vi "CPP-FIDpulseResponse.vi"() -> (5 "Plug in titles":string[](array[string]), 7 "Plug in values":string[](array[string]))   [LabVIEW 2021]
uses:
  Globals/Meas_global.vi
  <vilib>/measure/NI_MAPro.lvlib
  <vilib>/measure/mascope.llb/Transition Measurements N chan.vi
  <vilib>/measure/mascope.llb/Pulse Measurements N chan.vi
  <vilib>/Waveform/WDTOps.llb/WDT Get Waveform Subset DBL.vi
  <vilib>/measure/mascope.llb/Amplitude and Levels N chan.vi
  <vilib>/Analysis/NI_AALBase.lvlib
  <vilib>/Analysis/baseanly.llb/Mean (DBL).vi
panel:
  out "Cropped Means":dbl[](array[numeric])
  out "Cropped Sum all graph":waveform(dbl)[](graph)
  out "Duration of pulses":dbl
  out "Cropped Sum(all)":dbl[](array[numeric]) format="%#.0f"
  out "Starts":dbl[](array[numeric])
  out "sum(all)":dbl[](array[numeric])
  out "names":string[](array[string])
  out "NupEdges":i16[](array[numeric])
  out "sum(90-90)":dbl[](array[numeric])
  out "sum(10-10)":dbl[](array[numeric])
  out "(90-90) Graph":waveform(dbl)[](graph)
  out "(10-10) Graph":waveform(dbl)[](graph)
  out "t(90-90)":dbl[](array[numeric]) format="%.1f"
  out "t(10-10)":dbl[](array[numeric]) format="%.1f"
  out "complete":dbl[](array[numeric])
  out "t(10)":dbl[](array[numeric]) format="%.2f"
  out "slope (ppm/s)":dbl[](array[numeric]) format="%_3f"
  out "t(90)":dbl[](array[numeric]) format="%.2f"
  out "period (s)":dbl[](array[numeric]) format="%.1f"
  out "pulse duration (s)":dbl[](array[numeric]) format="%.1f"
  out "amplitude (ppm)":dbl[](array[numeric]) format="%.3f"
  in  "Enum":enum16{"Eng Units", "Voltages"}(ring)
  out "XY Graph":cluster{"Time (s)":dbl[], "Voltage":dbl[]}[](graph)
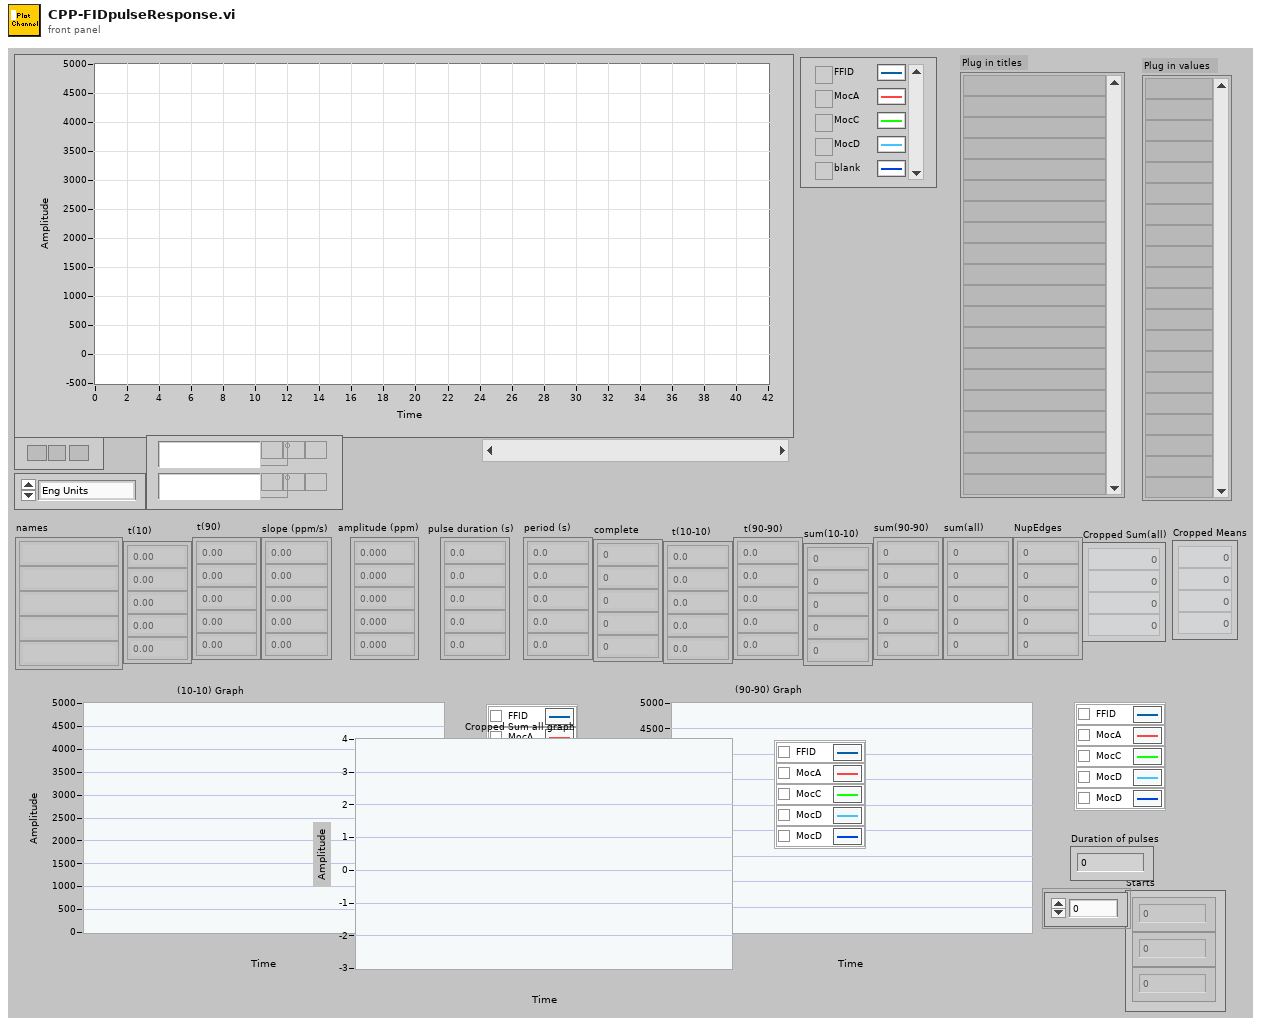
[diagram p1: front panel]
types:
  T1 = cluster{"method":enum32{"histogram", "peak", "auto select"}, "histogram size":i32, "histogram method":enum16{"mode"}, "reserved":dbl}
  T2 = cluster{"high ref level":dbl, "mid ref level":dbl, "low ref level":dbl, "ref units":u16}
  T3 = typedef "Analysis_info_cluster.ctl" = cluster{"Colour":u32, "Inst type":T4, "Inst name":string, "Symbol":string, "Code name":string, "Extra Info":string, "Inst Array":T5, "Extra Titles":string[], "Extra Values":string[], "U":dbl, "u^2":dbl, "u^3":dbl, "u^4":dbl, "Skew_u":dbl, "Kurt_u":dbl, "Sd Error in Mean":dbl, "% u'/U":dbl, "X":dbl, "Y":dbl, "Z":dbl, "Timescale integral Estimate":dbl, "Sd Error in Variance":dbl, "Calib File":path, "Calib Constants":dbl[], "Output Position":bool, "Stats":enum16{"None", "Basic", "Full"}, "Av Sampling Rate":dbl, "Av No of Samples":dbl, "Total Meas Time (s)":dbl, "ADAM Ch Name":string, "Max value":dbl, "Min value":dbl, "Req Sample Rate Hz":dbl, "Sync Delay Time (s)":dbl, "Ch No":i16, "Device":string, "Use Latest Calib":bool, "Port":string, "Metadata Ch Names":string[], "Metadata Ch Values":string[], "Label":string}
  T4 = typedef "Inst_type.ctl" = enum16{"Raw voltage", "Raw with zero offsetting", "Propeller anemometer", "Pressure Transducer", "Pitot-static tube", "Hot wire", "Cross wire 1", "Cross wire 2", "Generic Linear", "Generic Polynomial", "Generic BackPoly", "Fast FID", "Thermocouple", "Cold wire", "Pulsed Wire", "LDA Vel", "LDA Tran time", "LDA Arr time", "Microphone"}
  T5 = typedef "Instrument_Array.ctl" = enum16{"PWA", "LDA", "Analogue"}
  T6 = typedef "Time_Trace_Cluster.ctl" = cluster{"Weighting":dbl[], "Voltage":dbl[], "Eng Values":dbl[]}
  T7 = cluster{"start time":dbl, "end time":dbl, "ref levels":cluster{"high ref level":dbl, "mid ref level":dbl, "low ref level":dbl, "ref units":u16}}[]
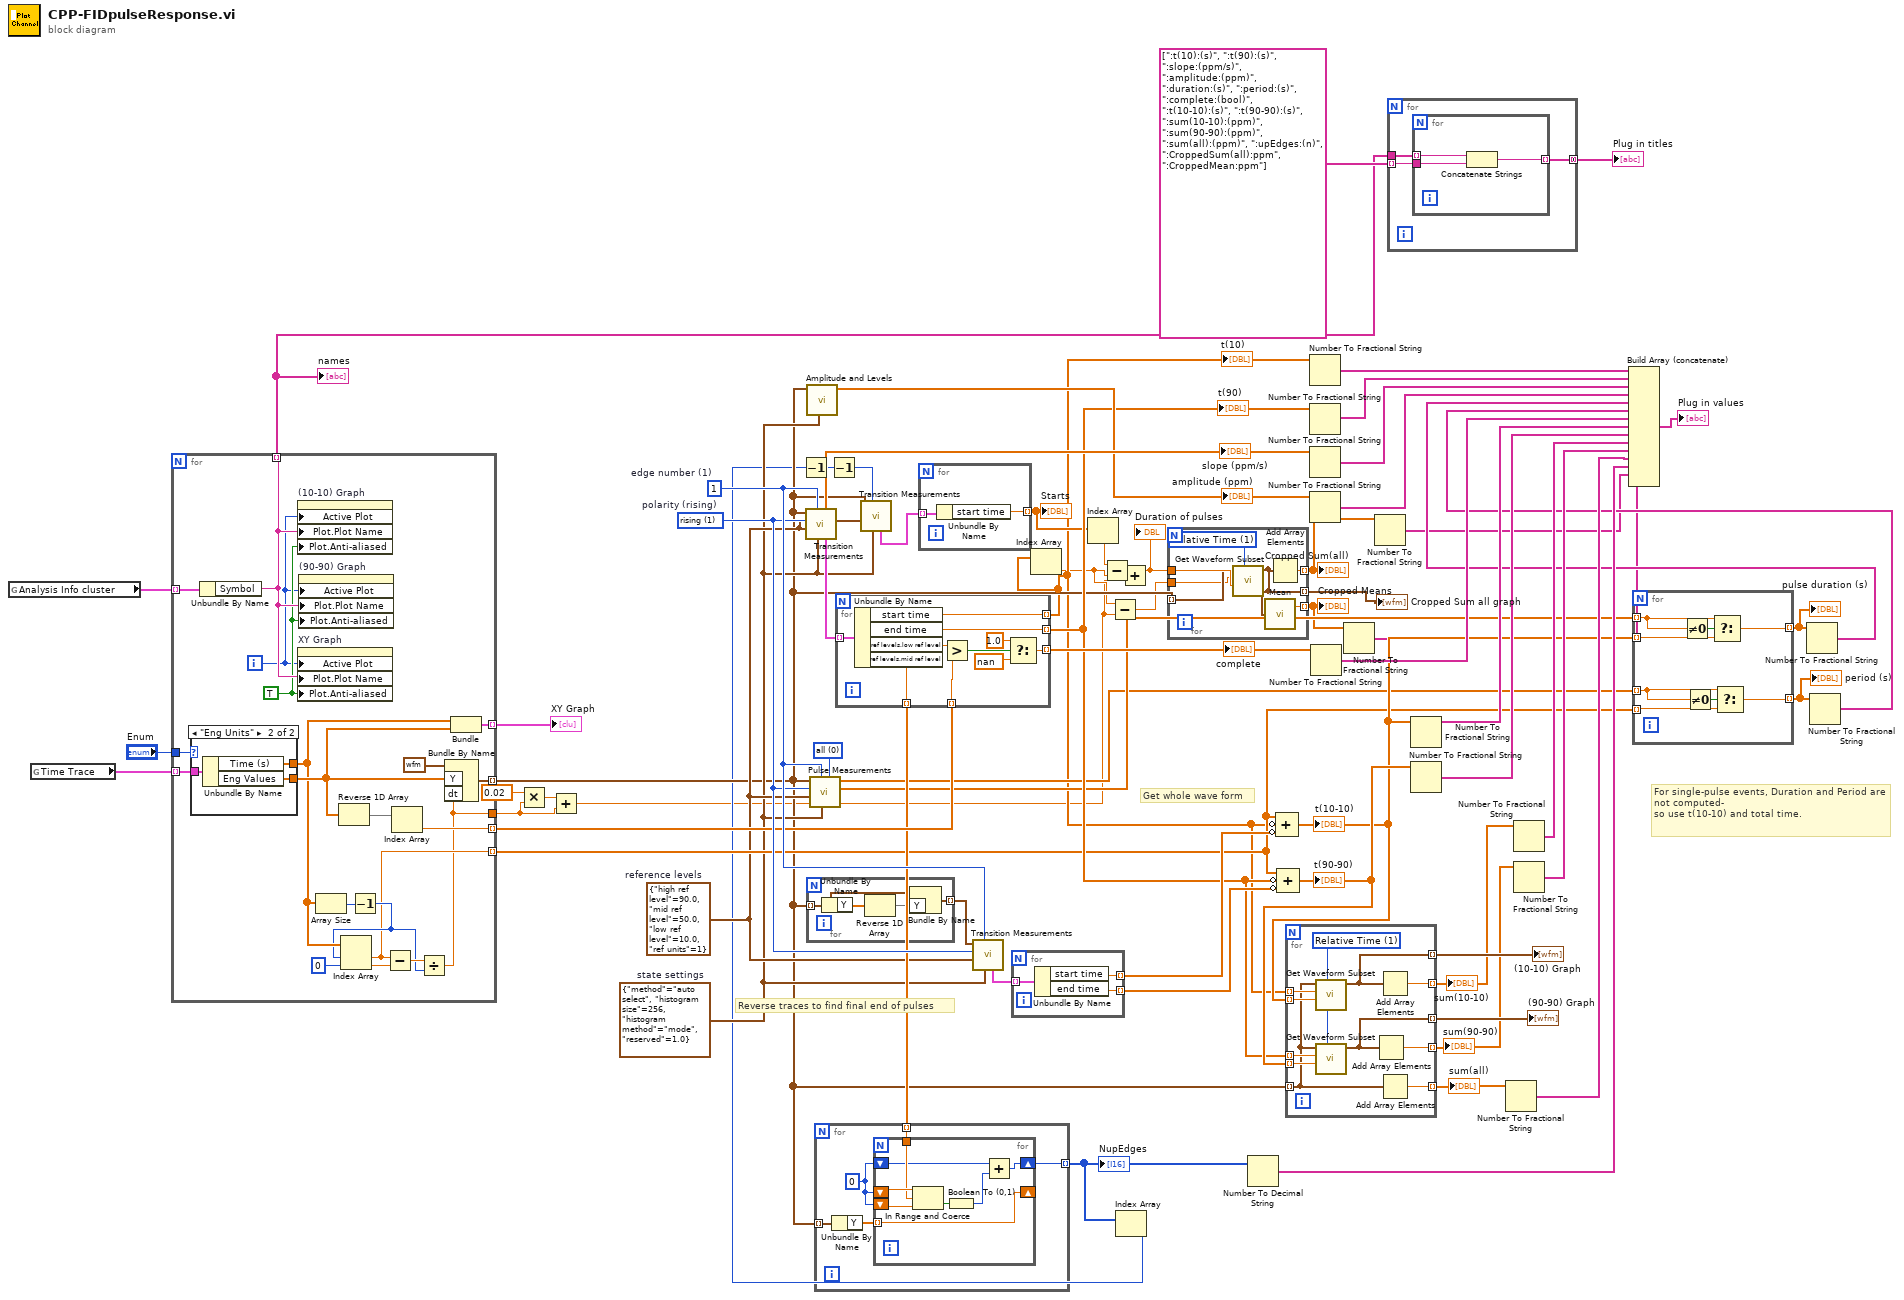
[diagram p0: block diagram]
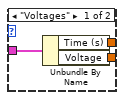
[diagram p2: hidden frame]
diagram:
  w54 = 1  # edge number (1)
  w53 = u16 1 items=["falling", "rising"]  # polarity (rising)
  w23 = T1 {"method"=enum."auto select", "histogram size"=256, "histogram method"=enum."mode", "reserved"=1.0}  # state settings
  w24 = T2 {"high ref level"=90.0, "mid ref level"=50.0, "low ref level"=10.0, "ref units"=1}  # reference levels
  w67 = u16 0 items=["all", "no period and duty cycle"] ("export mode")
  # "Get whole wave form"
  # "For single-pulse events, Duration and Period are not computed-\nso use t(10-10) and total time."
  # "Reverse traces to find final end of pulses"
  n1 = global read "Meas_global.vi" "Analysis Info cluster"() -> (w70:T3[])
  n2 = global read "Meas_global.vi" "Time Trace"() -> (w71:T6[])
  n3 = for {
    tunnel: w71 -> [w91] mode=indexing
    tunnel: [w90] -> w68 mode=indexing
    tunnel: w70 -> [w89] mode=indexing
    tunnel: "Enum" -> [w88]
    tunnel: [w87] -> w20 mode=indexing
    tunnel: [w76] -> w36 mode=indexing
    tunnel: [w84] -> w49 mode=indexing
    tunnel: [w77] -> w29 mode=indexing
    tunnel: [w72] -> w4
    i -> [w74]
    w75 = TRUE ("Plot.Anti-aliased")
    n4 = case shown="\"Eng Units\"" w88 {
      tunnel: [w94 w97] -> w85
      tunnel: [w93 w96] -> w82
      tunnel: w91 -> [w92 w95]
      frame "Voltages" {
        n5 = Unbundle By Name(w92) -> ("Time (s)"=w93:dbl[], "Voltage"=w94:dbl[])
      }
      frame "Eng Units" {
        n6 = Unbundle By Name(w95) -> ("Time (s)"=w96:dbl[], "Eng Values"=w97:dbl[])
      }
    }
    n7 = Unbundle By Name(w89) -> ("Symbol"=w76:string)
    n8 = property on="(10-10) Graph" class="WFGraph (strict)"("Active Plot"=w74, "Plot.Plot Name"=w76, "Plot.Anti-aliased"=w75) -> ()  [unwired: 2 in, 2 out]
    n9 = property on="XY Graph" class="XYGraph (strict)"("Active Plot"=w74, "Plot.Plot Name"=w76, "Plot.Anti-aliased"=w75) -> ()  [unwired: 2 in, 2 out]
    n10 = property on="(90-90) Graph" class="WFGraph (strict)"("Active Plot"=w74, "Plot.Plot Name"=w76, "Plot.Anti-aliased"=w75) -> ()  [unwired: 2 in, 2 out]
    n11 = Array Size(array=w82) -> (size(s)=w81:i32)
    n12 = Reverse 1D Array(array=w85) -> (reversed array=w86:dbl[])
    n13 = Decrement(x=w81) -> (x-1=w78:i32)
    n14 = Index Array(array=w82, index #1=w78, index #2=0 ("index")) -> (element #1=w77:dbl, element #2=w80:dbl)
    n15 = Subtract(x=w77, y=w80) -> (x-y=w83:dbl)
    n16 = Index Array(array=w86) -> (element=w84:dbl)  [unwired: 1 in]
    n17 = Divide(x=w83, y=w78) -> (x/y=w72:dbl)
    n18 = Bundle By Name(cluster=waveform(dbl) {"t0"=timestamp(0 s since 1904-01-01), "dt"=1.0, "Y"=[]} ("waveform"), "Y"=w85, "dt"=w72) -> (w87:waveform(dbl))
    n19 = Bundle("Time (s)"=w82, "Eng Values"=w85) -> (w90:cluster{"Time (s)":dbl[], "Eng Values":dbl[]})  [unwired: 1 in]
  }
  "XY Graph" <- w68
  "names" <- w36
  n20 = Multiply(x=0.02, y=w4) -> (x*y=w2:dbl)
  n21 = Add(x=w2, y=w4) -> (x+y=w1:dbl)
  n22 = call-poly <vilib>:"Transition Measurements.vi"("percent level settings"=w23, "edge number (1)"=w54, "reference levels"=w24, "polarity (rising)"=w53, "signal(s) in"=w20) -> ("measurement info"=w66:T7, "slope"=w61:dbl[])  [unwired: 1 in, 4 out]
  "slope (ppm/s)" <- w61
  n23 = call-poly <vilib>:"Amplitude and Levels.vi"("state settings"=w23, "signal(s) in"=w20) -> ("amplitude"=w58:dbl[])  [unwired: 6 in, 3 out]
  "amplitude (ppm)" <- w58
  n24 = for {
    tunnel: w20 -> [w98] mode=indexing
    tunnel: [w100] -> w52 mode=indexing
    n25 = Unbundle By Name(w98) -> ("Y"=w101:dbl[])
    n26 = Reverse 1D Array(array=w101) -> (reversed array=w99:dbl[])
    n27 = Bundle By Name(cluster=w98, "Y"=w99) -> (w100:waveform(dbl))
  }
  n28 = call-poly <vilib>:"Pulse Measurements.vi"("export mode"=w67, "percent level settings"=w23, "pulse number (1)"=w54, "reference levels"=w24, "polarity (high)"=w53, "signal(s) in"=w20) -> ("pulse duration"=w32:dbl[], "period"=w27:dbl[])  [unwired: 1 in, 3 out]
  n29 = for {
    tunnel: w66 -> [w111] mode=indexing
    tunnel: w49 -> [w106] mode=indexing
    tunnel: [w108] -> w56 mode=indexing
    tunnel: [w104] -> w40 mode=indexing
    tunnel: [w103] -> w17 mode=indexing
    tunnel: [w102] -> w37 mode=indexing
    n30 = Unbundle By Name(w111) -> ("start time"=w103:dbl, "end time"=w104:dbl, "ref levels.low ref level"=w110:dbl, "ref levels.mid ref level"=w102:dbl)
    n31 = Greater?(x=w110, y=w106) -> (0:w109:bool)
    n32 = Select(t=1.0, s=w109, f=nan) -> (s? t:f=w108:dbl)
  }
  "t(90)" <- w40
  "t(10)" <- w17
  "complete" <- w56
  n33 = for {
    tunnel: w20 -> [w113] mode=indexing
    tunnel: w37 -> [w116] mode=indexing
    tunnel: [w115] -> w16 mode=indexing
    w114 = i16 0
    n34 = Unbundle By Name(w113) -> ("Y"=w112:dbl[])
    n35 = for {
      shift-right: [w117] -> _
      shift-left: w114 -> [w124]
      shift-left: w114 -> [w123]
      tunnel: w116 -> [w122]
      shift-right: [w120] -> w115
      shift-left: w114 -> [w118]
      tunnel: w112 -> [w117] mode=indexing
      n36 = In Range and Coerce(upper limit=w124, x=w122, lower limit=w123) -> (In Range?=w121:bool)  [unwired: 1 out]
      n37 = Boolean To (0,1)(Boolean=w121) -> (0, 1=w119:i16)
      n38 = Add(x=w118, y=w119) -> (x+y=w120:i16)
    }
  }
  "NupEdges" <- w16
  n39 = call-poly <vilib>:"Transition Measurements.vi"("percent level settings"=w23, "edge number (1)"=w54, "reference levels"=w24, "polarity (rising)"=w53, "signal(s) in"=w52) -> ("measurement info"=w51:T7)  [unwired: 1 in, 5 out]
  n40 = for {
    tunnel: w51 -> [w127] mode=indexing
    tunnel: [w126] -> w50 mode=indexing
    tunnel: [w125] -> w48 mode=indexing
    n41 = Unbundle By Name(w127) -> ("start time"=w125:dbl, "end time"=w126:dbl)
  }
  n42 = Index Array(array=w17) -> (element=w13:dbl)  [unwired: 1 in]
  n43 = Subtract(x=w13, y=w1) -> (x-y=w12:dbl)
  n44 = Index Array(array=w16) -> (element=w15:i16)  [unwired: 1 in]
  n45 = Decrement(x=w15) -> (x-1=w8:i16)
  n46 = Decrement(x=w8) -> (x-1=w9:i16)
  n47 = call-poly <vilib>:"Transition Measurements.vi"("percent level settings"=w23, "edge number (1)"=w9, "reference levels"=w24, "signal(s) in"=w20) -> ("measurement info"=w22:T7)  [unwired: 2 in, 5 out]
  n48 = for {
    tunnel: w22 -> [w129] mode=indexing
    tunnel: [w128] -> w19 mode=indexing
    n49 = Unbundle By Name(w129) -> ("start time"=w128:dbl)
  }
  "Starts" <- w19
  n50 = Index Array(array=w19) -> (element=w18:dbl)  [unwired: 1 in]
  n51 = Subtract(x=w18, y=w13) -> (x-y=w21:dbl)
  n52 = Add(x=w21, y=w1) -> (x+y=w7:dbl)
  "Duration of pulses" <- w7
  n53 = for {
    tunnel: w7 -> [w136]
    tunnel: w20 -> [w135] mode=indexing
    tunnel: [w134] -> w11 mode=indexing
    tunnel: w12 -> [w133]
    tunnel: [w131] -> w14 mode=indexing
    tunnel: [w130] -> w6 mode=indexing
    w132 = u16 1 items=["Samples", "Relative Time"] ("start/duration format")
    n54 = call-poly <vilib>:"Get Waveform Subset.vi"("start/duration format"=w132, "duration"=w136, "start samples/time"=w133, "waveform in"=w135) -> ("waveform out"=w131:waveform(dbl))  [unwired: 2 in, 3 out]
    n55 = call-poly <vilib>:"Mean.vi"("X"=w131) -> ("mean"=w130:dbl)  [unwired: 1 out]
    n56 = Add Array Elements(numeric array=w131) -> (sum=w134:dbl)
  }
  "Cropped Sum(all)" <- w11
  "Cropped Sum all graph" <- w14
  "Cropped Means" <- w6
  n57 = Number To Decimal String(number=w16) -> (decimal integer string=w35:string[])  [unwired: 1 in]
  n58 = Compound Arithmetic op=ADD(w29, invert w17, invert w48) -> (w31:dbl[])
  "t(10-10)" <- w31
  n59 = Compound Arithmetic op=ADD(w29, invert w40, invert w50) -> (w47:dbl[])
  "t(90-90)" <- w47
  n60 = for {
    tunnel: w17 -> [w147] mode=indexing
    tunnel: w20 -> [w138] mode=indexing
    tunnel: w40 -> [w146] mode=indexing
    tunnel: w47 -> [w145] mode=indexing
    tunnel: w31 -> [w144] mode=indexing
    tunnel: [w142] -> w42 mode=indexing
    tunnel: [w140] -> w41 mode=indexing
    tunnel: [w141] -> w39 mode=indexing
    tunnel: [w139] -> w38 mode=indexing
    tunnel: [w137] -> w34 mode=indexing
    w143 = u16 1 items=["Samples", "Relative Time"] ("start/duration format")
    n61 = call-poly <vilib>:"Get Waveform Subset.vi"("start/duration format"=w143, "duration"=w144, "start samples/time"=w147, "waveform in"=w138) -> ("waveform out"=w142:waveform(dbl))  [unwired: 2 in, 3 out]
    n62 = call-poly <vilib>:"Get Waveform Subset.vi"("start/duration format"=w143, "duration"=w145, "start samples/time"=w146, "waveform in"=w138) -> ("waveform out"=w140:waveform(dbl))  [unwired: 2 in, 3 out]
    n63 = Add Array Elements(numeric array=w140) -> (sum=w139:dbl)
    n64 = Add Array Elements(numeric array=w142) -> (sum=w141:dbl)
    n65 = Add Array Elements(numeric array=w138) -> (sum=w137:dbl)
  }
  "(10-10) Graph" <- w42
  "(90-90) Graph" <- w41
  "sum(10-10)" <- w39
  "sum(90-90)" <- w38
  "sum(all)" <- w34
  n66 = Number To Fractional String(number=w17) -> (F-format string=w63:string[])  [unwired: 3 in]
  n67 = Number To Fractional String(number=w40) -> (F-format string=w60:string[])  [unwired: 3 in]
  n68 = Number To Fractional String(number=w61) -> (F-format string=w59:string[])  [unwired: 3 in]
  n69 = Number To Fractional String(number=w58) -> (F-format string=w57:string[])  [unwired: 3 in]
  n70 = Number To Fractional String(number=w56) -> (F-format string=w55:string[])  [unwired: 3 in]
  n71 = Number To Fractional String(number=w6) -> (F-format string=w5:string[])  [unwired: 3 in]
  n72 = Number To Fractional String(number=w11) -> (F-format string=w10:string[])  [unwired: 3 in]
  n73 = for {
    tunnel: w36 -> [w150]
    tunnel: string[] [":t(10):(s)", ":t(90):(s)", ":slope:(ppm/s)", ":amplitude:(ppm)", ":duration:(s)", ":period:(s)", ":complete:(bool)", ":t(10-10):(s)", ":t(90-90):(s)", ":sum(10-10):(ppm)", ":sum(90-90):(ppm)", ":sum(all):(ppm)", ":upEdges:(n)", ":CroppedSum(all):ppm", ":CroppedMean:ppm"] -> [w149] mode=indexing
    tunnel: [w148] -> w64 mode=concatenating
    n74 = for {
      tunnel: w150 -> [w153] mode=indexing
      tunnel: w149 -> [w152]
      tunnel: [w151] -> w148 mode=indexing
      n75 = Concatenate Strings(w153, w152) -> (w151:string)
    }
  }
  "Plug in titles" <- w64
  n76 = Number To Fractional String(number=w31) -> (F-format string=w46:string[])  [unwired: 3 in]
  n77 = Number To Fractional String(number=w47) -> (F-format string=w45:string[])  [unwired: 3 in]
  n78 = Number To Fractional String(number=w34) -> (F-format string=w33:string[])  [unwired: 3 in]
  n79 = Number To Fractional String(number=w39) -> (F-format string=w44:string[])  [unwired: 3 in]
  n80 = Number To Fractional String(number=w38) -> (F-format string=w43:string[])  [unwired: 3 in]
  n81 = for {
    tunnel: w32 -> [w160] mode=indexing
    tunnel: w31 -> [w159] mode=indexing
    tunnel: w29 -> [w158] mode=indexing
    tunnel: w27 -> [w156] mode=indexing
    tunnel: [w155] -> w25 mode=indexing
    tunnel: [w154] -> w26 mode=indexing
    n82 = Not Equal To 0?(x=w160) -> (x != 0?=w161:bool)
    n83 = Not Equal To 0?(x=w156) -> (x != 0?=w157:bool)
    n84 = Select(t=w160, s=w161, f=w159) -> (s? t:f=w155:dbl)
    n85 = Select(t=w156, s=w157, f=w158) -> (s? t:f=w154:dbl)
  }
  "pulse duration (s)" <- w25
  "period (s)" <- w26
  n86 = Number To Fractional String(number=w25) -> (F-format string=w30:string[])  [unwired: 3 in]
  n87 = Number To Fractional String(number=w26) -> (F-format string=w28:string[])  [unwired: 3 in]
  n88 = Build Array (concatenate)(w63, w60, w59, w57, w30, w28, w55, w46, w45, w44, w43, w33, w35, w10, w5) -> (→"Plug in values":string[])
